vi "FTW-ERR-PrependExplanation.vi"(7 "Exception Information":string, 11 "error in":errorcluster) -> (15 "error out":errorcluster)   [LabVIEW 2015]
panel:
  # "Inputs"
  # "Outputs"
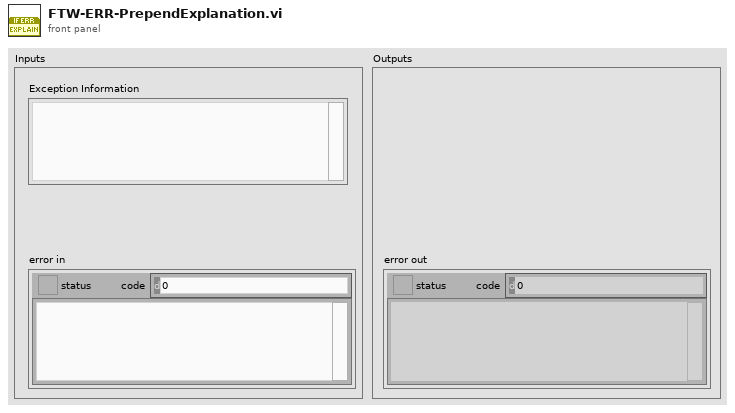
[diagram p1: front panel]
types:
  T1 = typedef "FTW-ERR-ExceptionType.ctl" = enum16{"No Error", "Error", "Warning"}
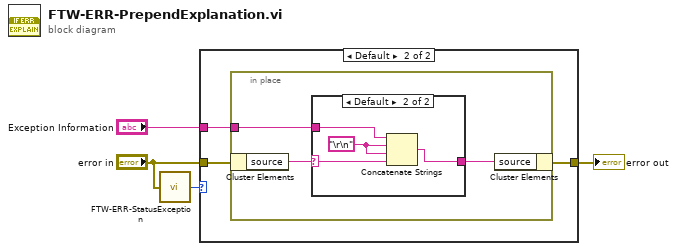
[diagram p0: block diagram]
diagram:
  n1 = call "FTW-ERR-StatusException.vi"("error to check"="error in") -> ("Exception"=w1:T1)
  n2 = case shown="Default" w1 {
    tunnel: [w5 w8] -> w4
    tunnel: "Exception Information" -> [_ w7]
    tunnel: "error in" -> [w5 w6]
    frame "No Error" {
    }
    frame Default {
      n3 = in-place {
        in-place-border: w7 -> [w10]
        n4 = in-place-cluster #1(w6) -> ("source"=w9:string)
        n5 = case shown="Default" w9 {
          selector: w9 -> [_ w15]
          tunnel: [w12 w16] -> w11
          tunnel: w10 -> [w12 w14]
          frame "" {
          }
          frame Default {
            w13 = "\r\n"
            n6 = Concatenate Strings(w14, w13, w13, w15) -> (w16:string)
          }
        }
        n7 = in-place-cluster #1("source"=w11) -> (w8:errorcluster)
      }
    }
  }
  "error out" <- w4
